vi "Read Debug Data.vi"(8 "error in (no error)":errorcluster, 11 "Debugger in":refnum<class "Debugger.lvclass">) -> (0 "error out":errorcluster, 3 "Debugger out":refnum<class "Debugger.lvclass">)   [LabVIEW 2020, in "Debugger.lvclass"]
uses:
  Debugger.lvclass
  TypeDefs/Debug Data.ctl
  Debugger.lvclass/Debugger.ctl
  <vilib>/Utility/miscctls.llb/LVMapReplaceAction.ctl
  465f6fcc-c403-4fca-a572-ae03f26762a0.vi
panel:
  out "output cluster":T1
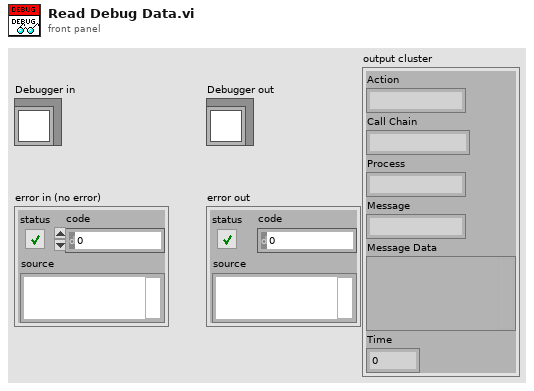
[diagram p1: front panel]
types:
  T1 = typedef "Debugger.lvclass/Debug Data.ctl" = cluster{"Action":string, "Call Chain":string, "Process":string, "Message":string, "Message Data":variant, "Time":u32}
  T2 = typedef "LVMapReplaceAction.ctl" = enum32{"Modify Entry only if found", "Add or Modify Entry", "Delete Entry"}
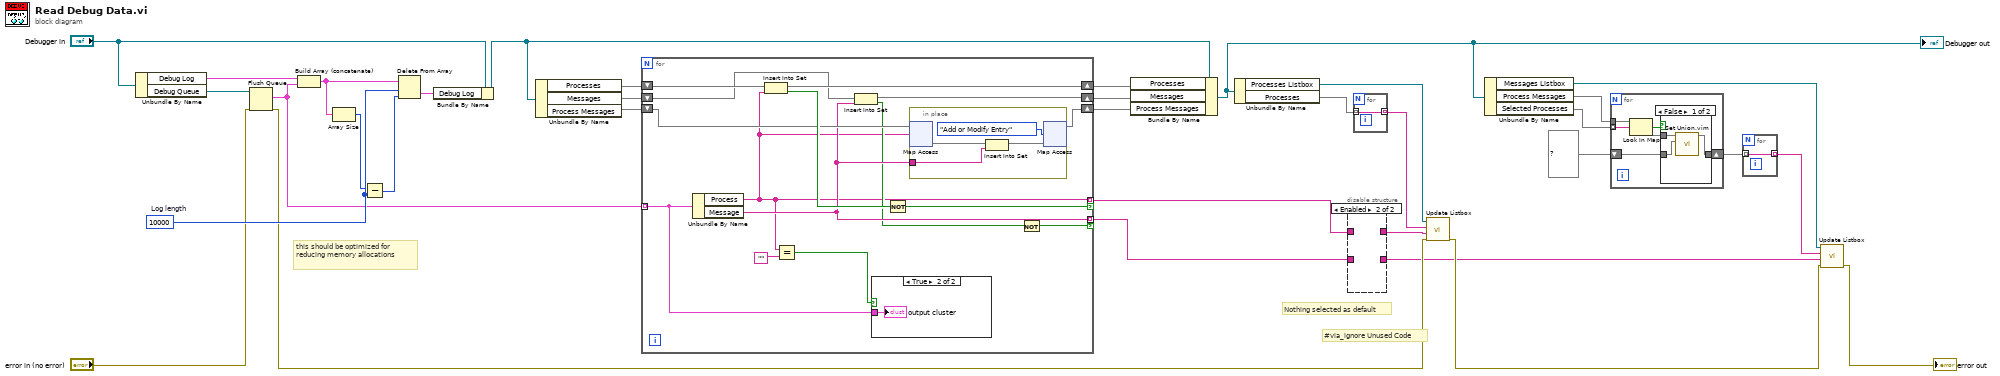
[diagram p0: block diagram]
diagram:
  w33 = 10000  # Log length
  # "#via_ignore Unused Code"
  # "Nothing selected as default"
  # "this should be optimized for reducing memory allocations"
  n1 = Unbundle By Name("Debugger in") -> ("Debug Log"=w29:T1[], "Debug Queue"=w27:refnum<queue>)
  n2 = Flush Queue(queue=w27, error in (no error)="error in (no error)") -> (remaining elements=w25:T1[], error out=w15:errorcluster)  [unwired: 1 out]
  n3 = Build Array (concatenate)(w29, w25) -> (w30:T1[])
  n4 = Array Size(array=w30) -> (size(s)=w31:i32)
  n5 = Subtract(x=w31, y=w33) -> (x-y=w32:i32)
  n6 = Delete From Array(array=w30, length=w33, index=w32) -> (deleted portion=w34:T1[])  [unwired: 1 out]
  n7 = Bundle By Name(cluster="Debugger in", "Debug Log"=w34) -> (w24:refnum<class "Debugger.lvclass">)
  n8 = Unbundle By Name(w24) -> ("Processes"=w23:set{string}, "Messages"=w6:set{string}, "Process Messages"=w12:map{string, set{string}})
  n9 = for {
    tunnel: w25 -> [w35] mode=indexing
    shift-right: [w48] -> w22
    shift-left: w23 -> [w49]
    tunnel: [w38] -> w3 mode=indexing if=w46
    tunnel: [w41] -> w1 mode=indexing if=w45
    shift-right: [w43] -> w11
    shift-left: w12 -> [w44]
    shift-right: [w40] -> w5
    shift-left: w6 -> [w42]
    n10 = Unbundle By Name(w35) -> ("Process"=w38:string, "Message"=w41:string)
    n11 = Insert Into Set(10:w38, 11:w49) -> (2:w47:bool, 3:w48:set{string})
    n12 = Equal?(x=w38, y="" ("Empty String Constant")) -> (x = y?=w36:bool)
    n13 = Insert Into Set(10:w41, 11:w42) -> (2:w39:bool, 3:w40:set{string})
    n14 = case shown="True" w36 {
      tunnel: w35 -> [_ w50]
      frame False {
      }
      frame True {
        "output cluster" <- w50
      }
    }
    n15 = Not(x=w47) -> (.not. x?=w46:bool)
    n16 = in-place "In Place Element Structure" {
      in-place-border: w41 -> [w51]
      n17 = in-place-map #1(w44, w38) -> (w54:set{string})  [unwired: 1 in, 1 out]
      n18 = Insert Into Set(10:w51, 11:w54) -> (3:w53:set{string})  [unwired: 1 out]
      n19 = in-place-map #1(w53, LVMapReplaceAction."Add or Modify Entry" ("action")) -> (w43:map{string, set{string}})  [unwired: 2 out]
    }
    n20 = Not(x=w39) -> (.not. x?=w45:bool)
  }
  n21 = Bundle By Name(cluster=w24, "Processes"=w22, "Messages"=w5, "Process Messages"=w11) -> (w16:refnum<class "Debugger.lvclass">)
  "Debugger out" <- w16
  n22 = Unbundle By Name(w16) -> ("Processes Listbox"=w21:refnum<vi>, "Processes"=w19:set{string})
  n23 = disable-structure "Diagram Disable Structure" shown="Enabled" {
    disable-tunnel: [w56 _] -> w4
    disable-tunnel: w3 -> [w56 _]
    disable-tunnel: [w55 _] -> w2
    disable-tunnel: w1 -> [w55 _]
    frame Disabled {
    }
    frame Enabled {
    }
  }
  n24 = for {
    tunnel: [w57] -> w20 mode=indexing
    tunnel: w19 -> [w57] mode=indexing
  }
  n25 = call "Update Listbox.vi"("error in (no error)"=w15, "New Items"=w4, "All Items"=w20, "ListBox in"=w21) -> ("error out"=w14:errorcluster)  [unwired: 7 in]
  n26 = Unbundle By Name(w16) -> ("Messages Listbox"=w17:refnum<vi>, "Process Messages"=w9:map{string, set{string}}, "Selected Processes"=w10:set{string})
  n27 = for {
    tunnel: w10 -> [w62] mode=indexing
    tunnel: w9 -> [w63]
    shift-right: [w59] -> w7
    shift-left: set{string} {} ("value") -> [w60]
    n28 = Look In Map(map=w63, key=w62) -> (key not found?=w58:bool, value=w61:set{string})  [unwired: 1 in]
    n29 = case shown="False" w58 {
      tunnel: w61 -> [w66 _]
      tunnel: w60 -> [w65 w67]
      tunnel: [w64 w67] -> w59
      frame False {
        n30 = call "Set Union.vim"("set 2"=w65, "set 1"=w66) -> ("union"=w64:set{string})  [unwired: 9 in]
      }
      frame True {
      }
    }
  }
  n31 = for {
    tunnel: [w68] -> w18 mode=indexing
    tunnel: w7 -> [w68] mode=indexing
  }
  n32 = call "Update Listbox.vi"("error in (no error)"=w14, "New Items"=w2, "All Items"=w18, "ListBox in"=w17) -> ("error out"=→"error out":errorcluster)  [unwired: 7 in]
